vi "receiver.vi"() -> ()   [LabVIEW 2009]
uses:
  Robot Status.ctl
  UDP Lib/UDP Network Location.ctl
  <vilib>/Platform/TimedLoop/XDataNode/XDataNode.xnode
  <vilib>/Platform/TimedLoop/XDataNode/loadlvalarms.vi
  <vilib>/Platform/TimedLoop/XDataNode/timing_clust.ctl
  <vilib>/Platform/TimedLoop/XDataNode/nitl_modes.ctl
  <vilib>/Platform/TimedLoop/XDataNode/wakeup.ctl
  <vilib>/Platform/TimedLoop/XDataNode/XDNodeRunTimeDep.lvlib
panel:
  out "Network Location":T1
  in  "stop":bool
  out "Status out":T2
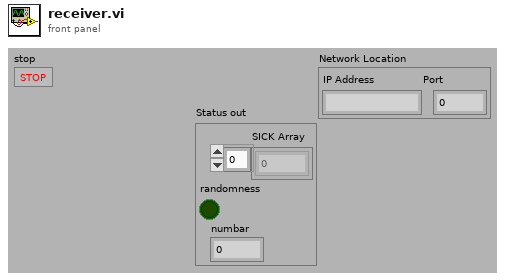
[diagram p1: front panel]
types:
  T1 = typedef "UDP Network Location.ctl" = cluster{"IP Address":string, "Port":u16}
  T2 = typedef "Robot Status.ctl" = cluster{"SICK Array":dbl[], "randomness":bool, "numbar":dbl}
  T3 = typedef "UDP Base.ctl" = cluster{"UDP Session":refnum<k16>, "UDP Socket Params":T4}
  T4 = typedef "UDP Socket Params.ctl" = cluster{"Local Port":u16, "Read Timeout":i32, "Write Timeout":i32}
  T5 = typedef "XDNodeRunTimeDep.lvlib/timing_clust.ctl" = cluster{"Expected End [f-1]":u64, "Actual End [f-1]":u64, "Finished Late? [f-1]":bool, "Expected End [i-1]":u64, "Actual End [i-1]":u64, "Finished Late? [i-1]":bool, "Expected Start [i]":u64, "Actual Start [i]":u64, "Expected Start [f]":u64, "Actual Start [f]":u64, "Source Name":string, "Structure Name":string, "Period":i64, "Deadline":i64, "Offset":i64, "Start":i64, "Priority":i32, "Timeout":i32, "Mode":T6, "Wakeup Reason":T7, "Error":errorcluster, "Source Type":string, "Secondary Source Type":string, "Global End Time":u64, "Global Start Time":u64, "Frame Duration":u64, "Iteration Duration":u64, "Assigned CPU":i32, "I/O Scan Engine Mode":u32}
  T6 = typedef "XDNodeRunTimeDep.lvlib/nitl_modes.ctl" = enum32{"No Change", "Process missed periods, maintain original phase", "Discard missed periods, maintain original phase", "Process missed periods, ignore original phase", "Discard missed periods, ignore original phase"}
  T7 = typedef "XDNodeRunTimeDep.lvlib/wakeup.ctl" = enum32{"Normal", "Aborted", "Asynchronous wakeup", "Timing source error", "Timed loop error", "Timeout"}
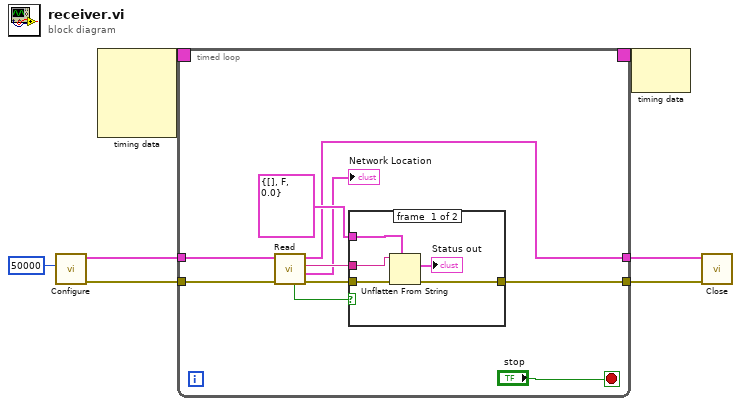
[diagram p0: block diagram]
diagram:
  n1 = call "Configure.vi"("Local Port"=u16 50000) -> ("error out"=w2:errorcluster, "UDP Base out"=w3:T3)  [unwired: 9 in]
  n2 = node-c288() -> (w7:T5)  [unwired: 4 in]
  n3 = timed-loop {
    timing: w7 -> [_]
    timing-out: [_] -> w6
    tunnel: [w14] -> w5
    tunnel: [w11] -> w4
    tunnel: w3 -> [w15]
    tunnel: w2 -> [w13]
    stop <- "stop" stop-if-true
    n4 = call "Read.vi"("error in (no error)"=w13, "UDP Base in"=w15) -> ("error out"=w12:errorcluster, "Network Location"=→"Network Location":T1, "Receive Data"=w16:string, "UDP Base out"=w14:T3, "Timeout"=w10:bool)  [unwired: 4 in, 1 out]
    n5 = case shown="False" w10 {
      tunnel: T2 {"SICK Array"=[], "randomness"=FALSE, "numbar"=0.0} ("Status out") -> [w22 _]
      tunnel: w16 -> [w21 _]
      tunnel: w12 -> [w20 w23]
      tunnel: [w19 w23] -> w11
      frame #0 {
        n6 = Unflatten From String(type=w22, binary string=w21, error in (no error)=w20) -> (value=→"Status out":T2, error out=w19:errorcluster)  [unwired: 2 in, 1 out]
      }
      frame #1 {
      }
    }
  }
  n7 = node-c288(w6) -> ()  [unwired: 1 out]
  n8 = call "Close.vi"("error in (no error)"=w4, "Cluster of class private data"=w5) -> ()  [unwired: 9 in, 1 out]
